vi "BRig_dataTrial_Cue2_I_HighProbSel.vi"() -> (2 "output_Cue2_I_HighProbSel":i32)   [LabVIEW 2014]
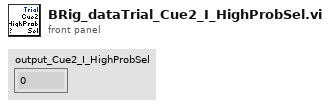
[diagram p1: front panel]
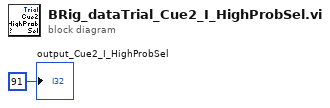
[diagram p0: block diagram]
diagram:
  "output_Cue2_I_HighProbSel" <- 91 ("output_iBlock")
